vi "Capture@UpdateImage__Parameter.vi"(1 "ParamterIn":string) -> (0 "ParamterOut":string)   [LabVIEW 2020]
panel:
  in  "Interval":string(combo)
  in  "CamName":string(combo)
  in  "Confirm":bool
  # "Capture@UpdateImage $Capture(,$Interval)"
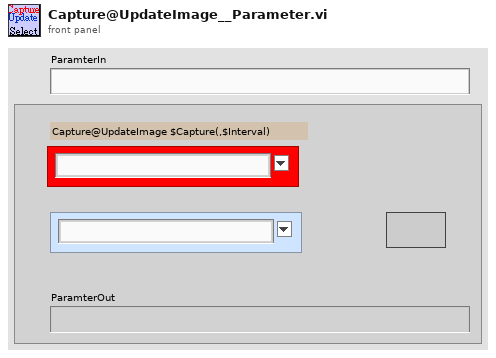
[diagram p1: front panel]
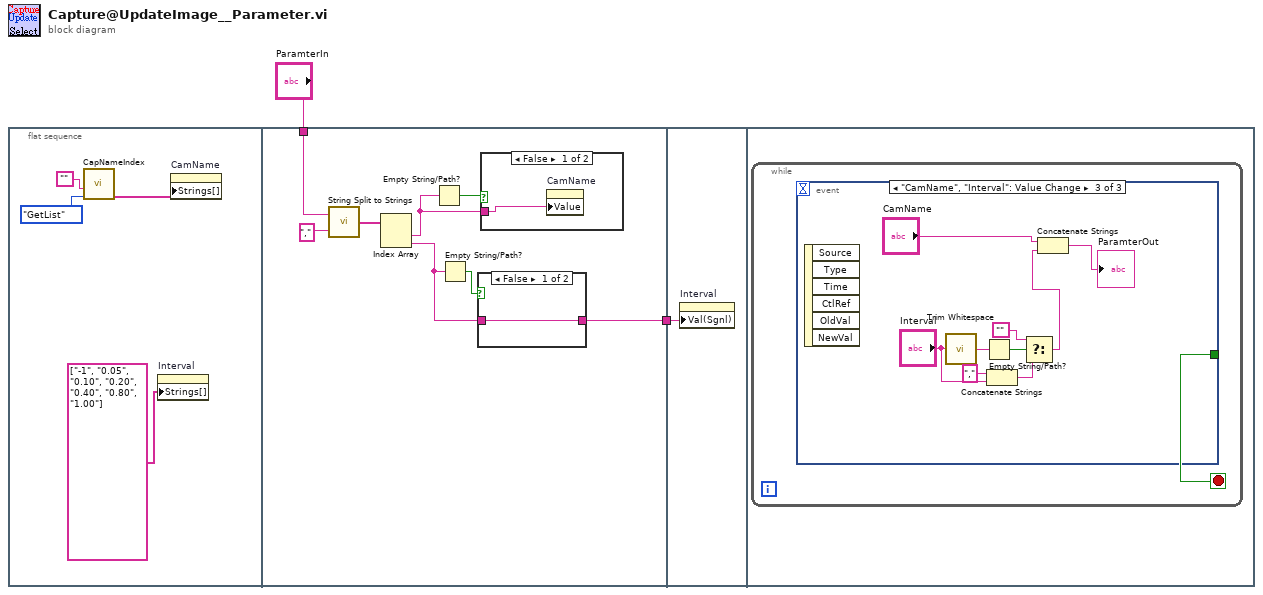
[diagram p0: block diagram]
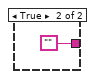
[diagram p2: hidden frame]
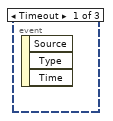
[diagram p4: hidden frame]
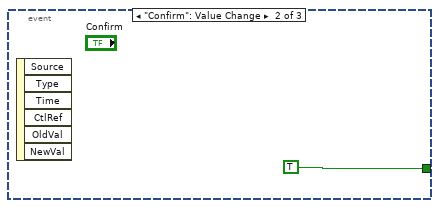
[diagram p5: hidden frame]
diagram:
  n1 = flat-sequence {
    tunnel: "ParamterIn" -> [w10]
    tunnel: [w7] -> w1
    tunnel: w1 -> [w18]
    frame #0 {
      n2 = call "CapNameIndex.vi"("OP"=enum16{"AddCam", "GetIndex", "Init", "GetList"}."GetList", "CamName"="") -> ("DeviceList"=w5:string[])  [unwired: 2 in, 3 out]
      n3 = property on="Interval" class="CmbBox"("Strings[]"=string[] ["-1", "0.05", "0.10", "0.20", "0.40", "0.80", "1.00"] ("Strings []")) -> ()  [unwired: 2 in, 2 out]
      n4 = property on="CamName" class="CmbBox"("Strings[]"=w5) -> ()  [unwired: 2 in, 2 out]
    }
    frame #1 {
      n5 = call "String Split to Strings.vi"("search string/char (-)"=",", "String"=w10) -> ("Array"=w11:string[])
      n6 = Index Array(array=w11) -> (element #1=w9:string, element #2=w8:string)  [unwired: 2 in]
      n7 = Empty String/Path?(string/path=w9) -> (empty?=w14:bool)
      n8 = Empty String/Path?(string/path=w8) -> (empty?=w13:bool)
      n9 = case shown="False" w13 {
        tunnel: [w15 ""] -> w7
        tunnel: w8 -> [w15 _]
        frame False {
        }
        frame True {
        }
      }
      n10 = case shown="False" w14 {
        tunnel: w9 -> [w17 _]
        frame False {
          n11 = property on="CamName" class="CmbBox"("Value"=w17) -> ()  [unwired: 2 in, 2 out]
        }
        frame True {
        }
      }
    }
    frame #2 {
      n12 = property on="Interval" class="CmbBox"("Val(Sgnl)"=w18) -> ()  [unwired: 2 in, 2 out]
    }
    frame #3 {
      n13 = while {
        stop <- w19 stop-if-true
        n14 = event shown="[2] \"CamName\", \"Interval\": Value Change" {
          selector: _ -> [_ _ _]
          dyn-events: _ -> [_ _ _]
          timeout: _ -> [_ _ _]
          tunnel: [_ TRUE _] -> w19
          event Timeout {
            n15 = event-data() -> ()  [unwired: 1 in, 3 out]
          }
          event "Confirm": Value Change {
            n16 = event-data() -> ()  [unwired: 1 in, 6 out]
          }
          event "CamName", "Interval": Value Change {
            n17 = event-data() -> ()  [unwired: 1 in, 6 out]
            n18 = call <vilib>:"Trim Whitespace.vi"("string"="Interval") -> ("trimmed string"=w24:string)  [unwired: 1 in]
            n19 = Empty String/Path?(string/path=w24) -> (empty?=w25:bool)
            n20 = Concatenate Strings("," ("string"), "Interval") -> (w27:string)
            n21 = Select(t="", s=w25, f=w27) -> (s? t:f=w22:string)
            n22 = Concatenate Strings("CamName", w22) -> (→"ParamterOut":string)
          }
        }
      }
    }
  }
